vi "Convert Unscaled to Scaled.vi"(2 "Unscaled Data":i32[][](array[numeric]), 3 "Header Information":dbl[][](array[numeric])) -> (1 "Scaled Data":waveform(dbl)[](graph))   [LabVIEW 2013]
doc: "This subVI takes header information and unscaled data and performs a 1D polynomial evaluation to return the scaled data."
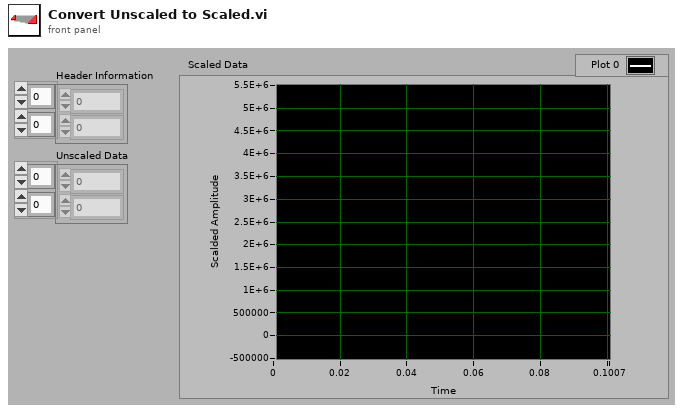
[diagram p1: front panel]
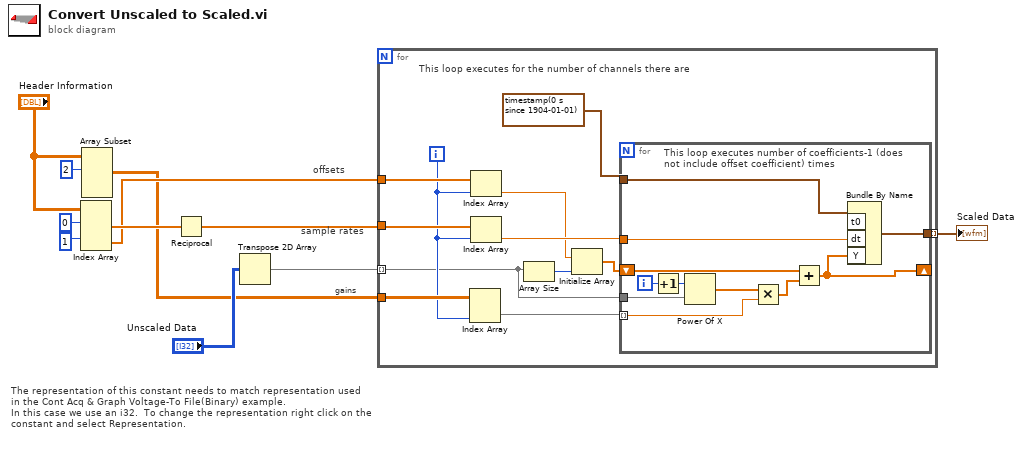
[diagram p0: block diagram]
diagram:
  # "The representation of this constant needs to match representation used\nin the Cont Acq & Graph Voltage-To File(Binary) example.\nIn this case we use an i32.  To change the representation right click on the\nconstant and select Representation."
  # "offsets"
  # "gains"
  # "sample rates"
  n1 = Index Array(array="Header Information", index (row) #1=0 ("index"), index (row) #2=1 ("index (row)")) -> (element #1=w8:dbl[], element #2=w6:dbl[])  [unwired: 2 in]
  n2 = Array Subset(array="Header Information", index (row)=2 ("index")) -> (w3:dbl[][])  [unwired: 3 in]
  n3 = Reciprocal(x=w8) -> (1/x=w5:dbl[])
  n4 = Transpose 2D Array(2D array="Unscaled Data") -> (transposed array=w4:i32[][])
  n5 = for {
    tunnel: w4 -> [w13] mode=indexing
    tunnel: w5 -> [w19]
    tunnel: w6 -> [w21]
    tunnel: w3 -> [w20]
    tunnel: [w16] -> w1 mode=indexing
    i -> [w17]
    # "This loop executes for the number of channels there are"
    n6 = Index Array(array=w20, index (col)=w17) -> (element=w23:dbl[])  [unwired: 1 in]
    n7 = Index Array(array=w21, index=w17) -> (element=w15:dbl)
    n8 = Index Array(array=w19, index=w17) -> (element=w18:dbl)
    n9 = Array Size(array=w13) -> (size(s)=w12:i32)
    n10 = Initialize Array(w15, w12) -> (w14:dbl[])
    n11 = for {
      shift-right: [w29] -> _
      shift-left: w14 -> [w24]
      tunnel: w23 -> [w33] mode=indexing
      tunnel: w18 -> [w32]
      tunnel: timestamp(0 s since 1904-01-01) ("t0") -> [w31]
      tunnel: [w30] -> w16
      tunnel: w13 -> [w28]
      i -> [w34]
      # "This loop executes number of coefficients-1 (does\nnot include offset coefficient) times"
      n12 = Increment(x=w34) -> (x+1=w27:i32)
      n13 = Power Of X(1:w28, 2:w27) -> (0:w26:dbl[])
      n14 = Multiply(x=w26, y=w33) -> (x*y=w25:dbl[])
      n15 = Add(x=w24, y=w25) -> (x+y=w29:dbl[])
      n16 = Bundle By Name("t0"=w31, "dt"=w32, "Y"=w29) -> (w30:waveform(dbl))  [unwired: 1 in]
    }
  }
  "Scaled Data" <- w1
